vi "Test Filter Test by Name with plus.vi"(8 "error in (no error)":errorcluster, 11 "Test Case In":refnum<class "Filter Test.lvclass">) -> (0 "error out":errorcluster, 3 "Test Case Out":refnum<class "Filter Test.lvclass">)   [LabVIEW 2020, in "Filter Test.lvclass"]
uses:
  Filter Test.lvclass
  C:/Program Files (x86)/National Instruments/LabVIEW 2020/vi.lib/Astemes/LUnit/Test Case.lvclass
  Test Doubles/Test Case Test Double/Test Case Test Double.lvclass
  <vilib>/Astemes/LUnit/Test Case.lvclass/Test Case.ctl
  5d80b200-0084-484b-a338-0aaa4416bded.vi
  <vilib>/Astemes/LUnit/Palette/Pass If.vi
  <vilib>/Astemes/LUnit/Append Fail Result.vi
  <vilib>/Astemes/LUnit/Append Pass Result.vi
  <vilib>/Astemes/LUnit/Run In UI.vi
  <vilib>/Utility/error.llb/Clear Errors.vi
  source/User Interface/Support/Filters/Filter/Filter.lvclass
  source/User Interface/Support/Filters/Static Filter/Static Filter.lvclass
  source/API/LUnit Test Suite/LUnit Test Suite.lvclass
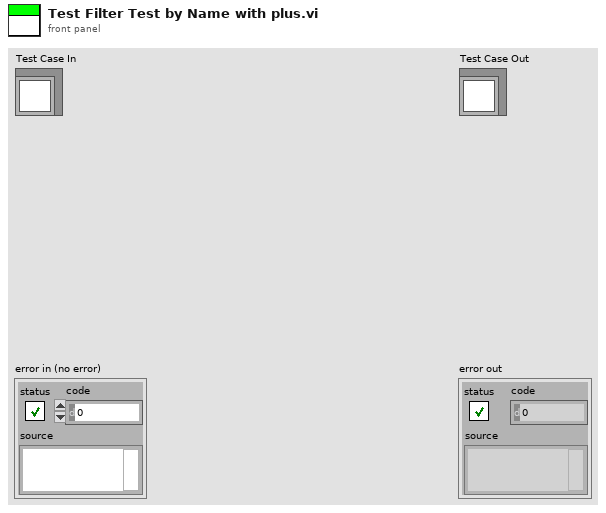
[diagram p1: front panel]
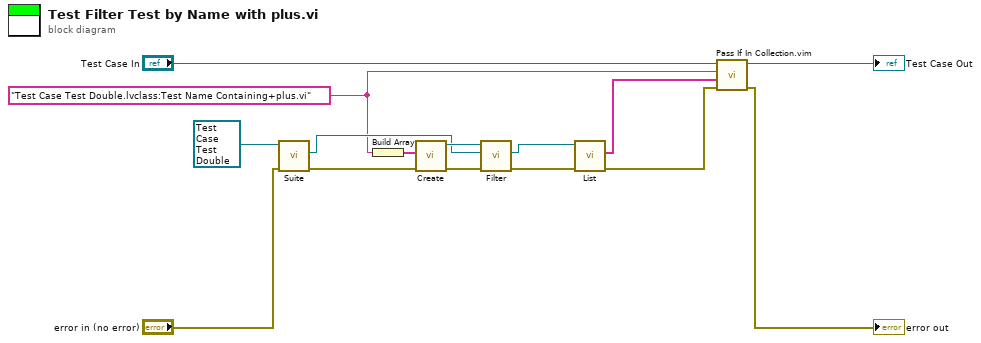
[diagram p0: block diagram]
diagram:
  w1 = "Test Case Test Double.lvclass:Test Name Containing+plus.vi"
  n1 = call-dynamic "Suite.vi"("error in (no error)"="error in (no error)", "Test Case Class in"=refnum<class "Test Case Test Double.lvclass"> refnum ("Test Case Test Double.lvclass")) -> ("error out"=w12:errorcluster, "LUnit Test Suite Out"=w4:refnum<class "LUnit Test Suite.lvclass">)  [unwired: 7 in, 1 out]
  n2 = Build Array(w1) -> (w2:string[])
  n3 = call "Create.vi"("error in (no error)"=w12, "Tests"=w2) -> ("error out"=w10:errorcluster, "Static Filter"=w11:refnum<class "Filter.lvclass">)  [unwired: 8 in]
  n4 = call-dynamic "Filter.vi"("error in (no error)"=w10, "Test Suite"=w4, "Filter in"=w11) -> ("error out"=w8:errorcluster, "Filtered Test Suite"=w9:refnum<class "LUnit Test Suite.lvclass">)  [unwired: 7 in]
  n5 = call "List.vi"("error in (no error)"=w8, "LUnit Test Suite In"=w9) -> ("error out"=w6:errorcluster, "List of Runnables"=w7:string[])  [unwired: 8 in]
  n6 = call "Pass If In Collection.vim"("error in (no error)"=w6, "Collection"=w7, "Expected Element"=w1, "LUnit Test Case In"="Test Case In") -> ("error out"=→"error out":errorcluster, "LUnit Test Case Out"=→"Test Case Out":refnum<class "Filter Test.lvclass">)  [unwired: 6 in]
